vi "readlabel.vi"(10 "ptr":u32, 11 "Buffer IN":string) -> (2 "Label":string, 3 "Buffer OUT":string)   [LabVIEW 2017, in "HEKAdat.lvclass"]
uses:
  HEKAdat.lvclass
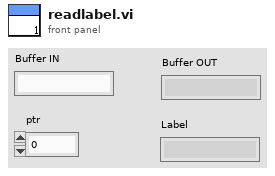
[diagram p1: front panel]
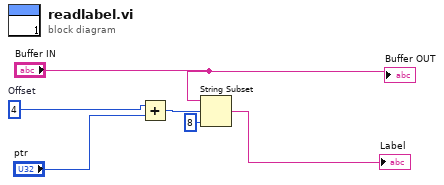
[diagram p0: block diagram]
diagram:
  w2 = u32 4  # Offset
  n1 = Add(x=w2, y="ptr") -> (x+y=w1:u32)
  n2 = String Subset(string="Buffer IN", offset (0)=w1, length (rest)=u32 8 ("length (rest)")) -> (substring=→"Label":string)
  "Buffer OUT" <- "Buffer IN"
